vi "LogicForUT.vi"(7 "Data Clusters":variant[](array[variant]), 8 "error in (no error)":errorcluster, 9 "Array":T1(array[cluster]), 10 "LV Data":T2, 11 "TableLogger_CSV_Actor in":refnum<class "TableLogger_CSV_Actor.lvclass">) -> (0 "error out":errorcluster, 1 "Selected?T":bool, 2 "Deleted?T":bool, 3 "Updated?T":bool)   [LabVIEW 2014, in "TableLogger_CSV_Actor.lvlib" / "TableLogger_CSV_Actor.lvclass"]
uses:
  TableLogger_CSV_Actor.lvclass
  TableLogger_CSV_Actor.lvclass/TableLogger_CSV_Actor.ctl
  <userlib>/_OpenG.lib/array/array.llb/Search 1D Array (String)__ogtk.vi
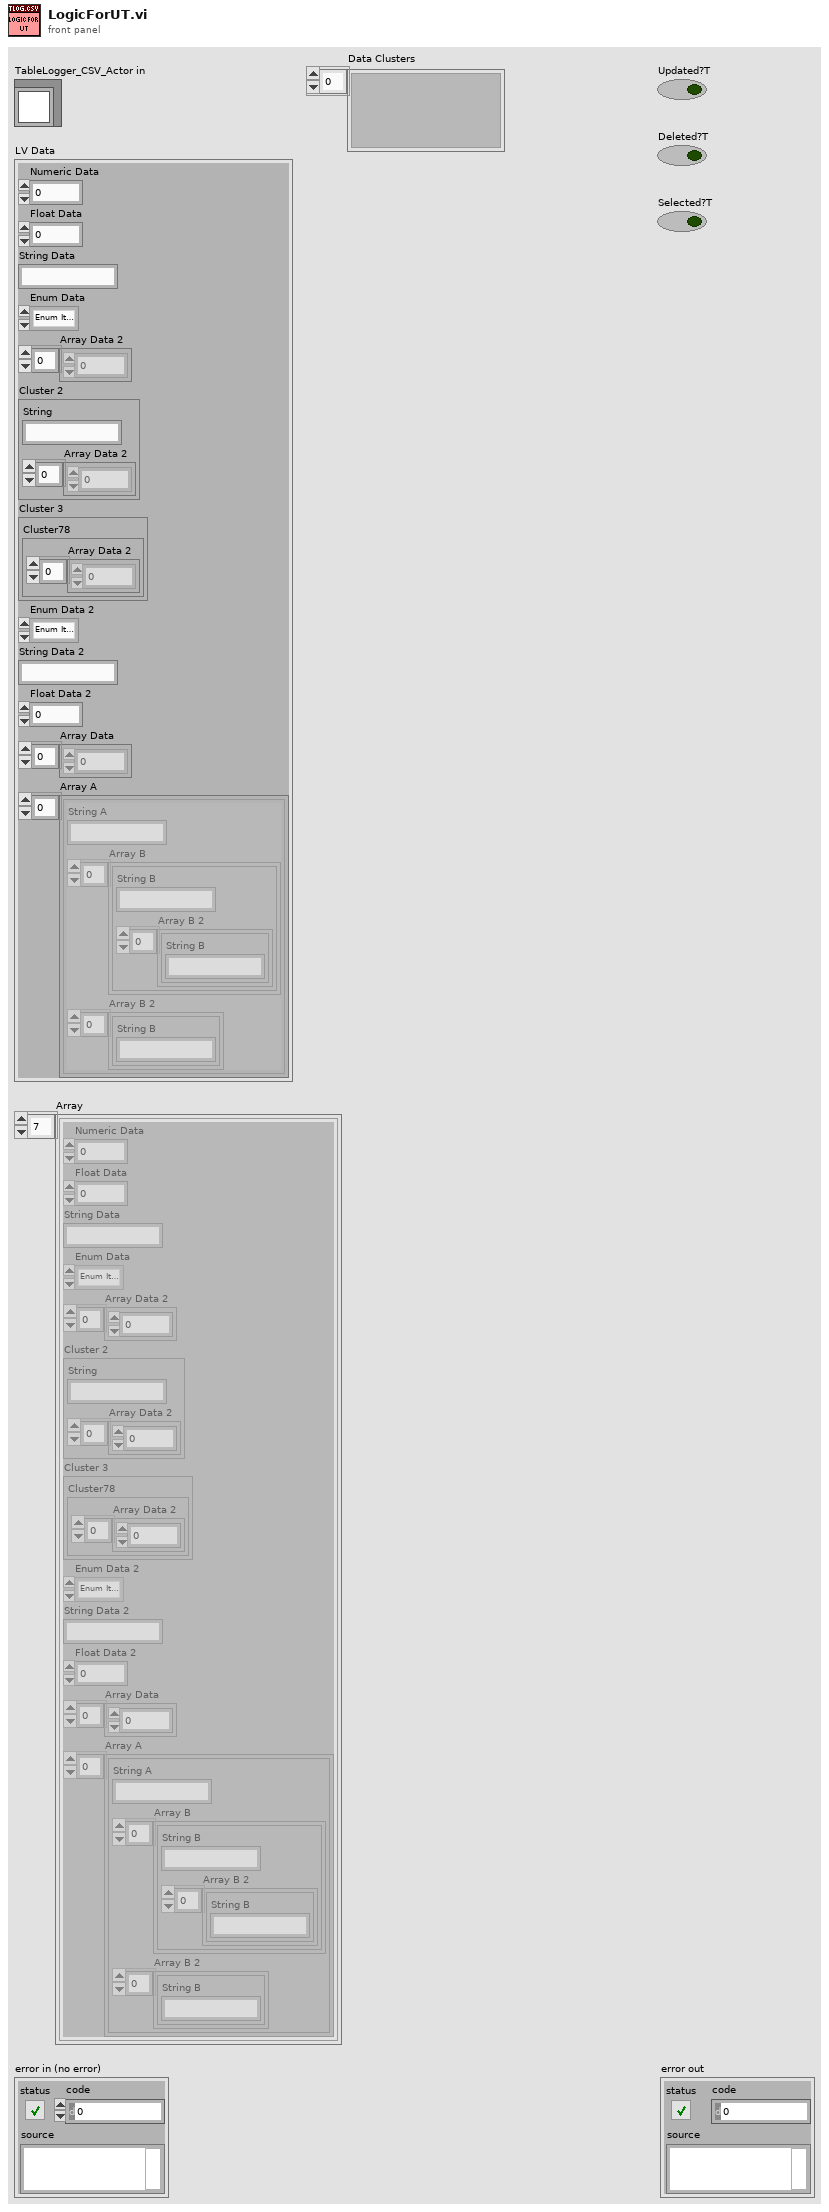
[diagram p1: front panel]
types:
  T1 = cluster{"Numeric Data":i32, "Float Data":dbl, "String Data":string, "Enum Data":enum16{"Enum Item 1", "Enum Item 2"}, "Array Data 2":i32[], "Cluster 2":cluster{"String":string, "Array Data 2":i32[]}, "Cluster 3":cluster{"Cluster78":cluster{"Array Data 2":i32[]}}, "Enum Data 2":enum16{"Enum Item 1", "Enum Item 2"}, "String Data 2":string, "Float Data 2":dbl, "Array Data":i32[], "Array A":cluster{"String A":string, "Array B":cluster{"String B":string, "Array B 2":cluster{"String B":string}[]}[], "Array B 2":cluster{"String B":string}[]}[]}[]
  T2 = cluster{"Numeric Data":i32, "Float Data":dbl, "String Data":string, "Enum Data":enum16{"Enum Item 1", "Enum Item 2"}, "Array Data 2":i32[], "Cluster 2":cluster{"String":string, "Array Data 2":i32[]}, "Cluster 3":cluster{"Cluster78":cluster{"Array Data 2":i32[]}}, "Enum Data 2":enum16{"Enum Item 1", "Enum Item 2"}, "String Data 2":string, "Float Data 2":dbl, "Array Data":i32[], "Array A":cluster{"String A":string, "Array B":cluster{"String B":string, "Array B 2":cluster{"String B":string}[]}[], "Array B 2":cluster{"String B":string}[]}[]}
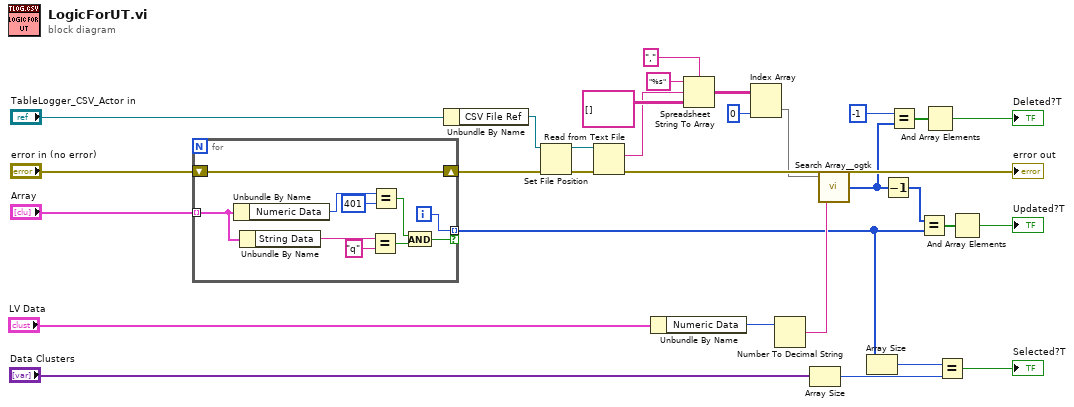
[diagram p0: block diagram]
diagram:
  n1 = for {
    tunnel: "Array" -> [w35] mode=indexing
    tunnel: [w32] -> w5 mode=indexing if=w33
    shift-right: [w31] -> w30
    shift-left: "error in (no error)" -> [w31]
    i -> [w32]
    n2 = Unbundle By Name(w35) -> ("Numeric Data"=w40:i32)
    n3 = Unbundle By Name(w35) -> ("String Data"=w37:string)
    n4 = Equal?(x=w37, y="q") -> (x = y?=w34:bool)
    n5 = Equal?(x=w40, y=401) -> (x = y?=w38:bool)
    n6 = And(x=w38, y=w34) -> (x .and. y?=w33:bool)
  }
  n7 = Unbundle By Name("TableLogger_CSV_Actor in") -> ("CSV File Ref"=w26:refnum<file>)
  n8 = Set File Position(refnum=w26, error in=w30) -> (refnum out=w12:refnum<file>, error out=w13:errorcluster)  [unwired: 2 in]
  n9 = Read from Text File(file (use dialog)=w12, error in=w13) -> (text=w14:string, error out=→"error out":errorcluster)  [unwired: 2 in, 2 out]
  n10 = Unbundle By Name("LV Data") -> ("Numeric Data"=w27:i32)
  n11 = Spreadsheet String To Array(delimiter (Tab)=",", format string="%s", spreadsheet string=w14, array type (2D Dbl)=string[][] []) -> (array=w18:string[][])
  n12 = Index Array(array=w18, index (col)=0 ("disabled index (col)")) -> (element=w20:string[])  [unwired: 1 in]
  n13 = Number To Decimal String(number=w27) -> (decimal integer string=w21:string)  [unwired: 1 in]
  n14 = Array Size(array="Data Clusters") -> (size(s)=w3:i32)
  n15 = call-poly <userlib>:"Search Array__ogtk.vi"("Array"=w20, "Element Data"=w21) -> ("Indices of Elements"=w9:i32[])  [unwired: 7 in]
  n16 = Array Size(array=w5) -> (size(s)=w4:i32)
  n17 = Decrement(x=w9) -> (x-1=w10:i32[])
  n18 = Equal?(x=-1 ("Numeric"), y=w9) -> (x = y?=w6:bool[])
  n19 = Equal?(x=w10, y=w5) -> (x = y?=w22:bool[])
  n20 = And Array Elements(Boolean array=w6) -> (logical AND=→"Deleted?T":bool)
  n21 = Equal?(x=w4, y=w3) -> (x = y?=→"Selected?T":bool)
  n22 = And Array Elements(Boolean array=w22) -> (logical AND=→"Updated?T":bool)
